vi "关键参数区.vi"(11 "数组":u16[](array[numeric]) format="%04xH") -> (3 "关键参数区":T1)   [LabVIEW 2016, in "斯坦道氨氮.lvlib"]
panel:
  # "共占用56 WORD"
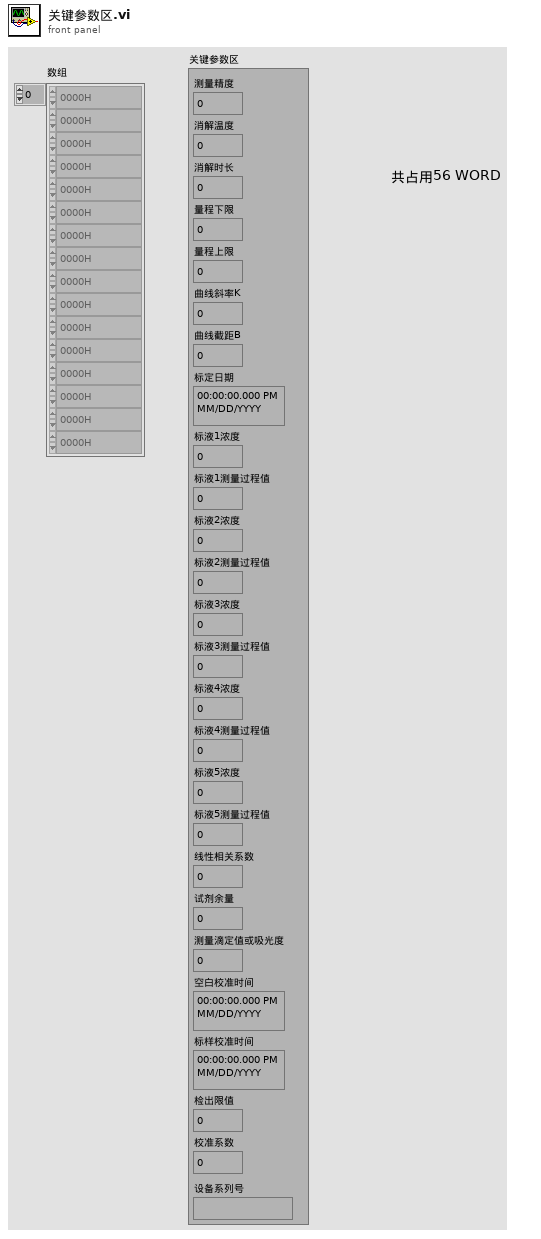
[diagram p1: front panel]
types:
  T1 = cluster{"测量精度":u16, "消解温度":u16, "消解时长":u16, "量程下限":sgl, "量程上限":sgl, "曲线斜率K":sgl, "曲线截距B":sgl, "标定日期":timestamp, "标液1浓度":sgl, "标液1测量过程值":sgl, "标液2浓度":sgl, "标液2测量过程值":sgl, "标液3浓度":sgl, "标液3测量过程值":sgl, "标液4浓度":sgl, "标液4测量过程值":sgl, "标液5浓度":sgl, "标液5测量过程值":sgl, "线性相关系数":sgl, "试剂余量":u32, "测量滴定值或吸光度":sgl, "空白校准时间":timestamp, "标样校准时间":timestamp, "检出限值":sgl, "校准系数":sgl, "设备系列号":string}
  T2 = cluster{"WORD":u16, "WORD":u16, "WORD":u16, "FLOAT":sgl, "FLOAT":sgl, "FLOAT":sgl, "FLOAT":sgl, "time stamp":timestamp, "FLOAT":sgl, "FLOAT":sgl, "FLOAT":sgl, "FLOAT":sgl, "FLOAT":sgl, "FLOAT":sgl, "FLOAT":sgl, "FLOAT":sgl, "FLOAT":sgl, "FLOAT":sgl, "FLOAT":sgl, "DWORD":i32, "FLOAT":sgl, "time stamp":timestamp, "time stamp":timestamp, "FLOAT":sgl, "FLOAT":sgl, "string":string}
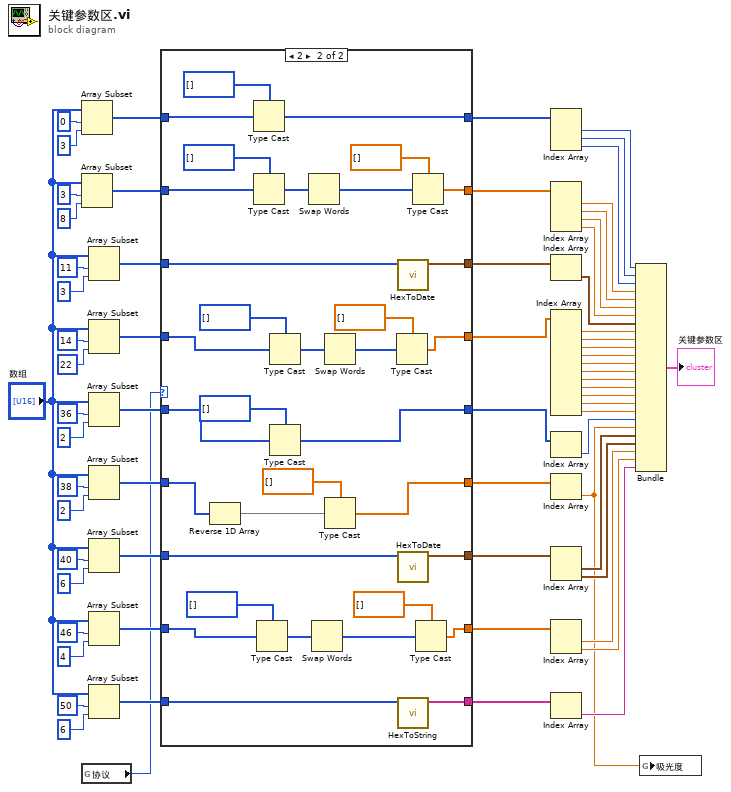
[diagram p0: block diagram]
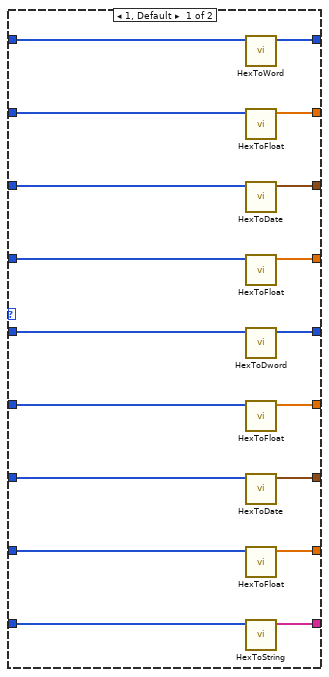
[diagram p2: hidden frame]
diagram:
  n1 = Array Subset(array="数组", index=0 ("索引"), length=3 ("长度")) -> (w60:u16[])
  n2 = Array Subset(array="数组", index=3 ("索引"), length=8 ("长度")) -> (w56:u16[])
  n3 = global read "总磷总氮断电保存全局变量.vi" "协议"() -> (w2:u16)
  n4 = Array Subset(array="数组", index=11 ("索引"), length=3 ("长度")) -> (w48:u16[])
  n5 = Array Subset(array="数组", index=14 ("索引"), length=22 ("长度")) -> (w43:u16[])
  n6 = Array Subset(array="数组", index=36 ("索引"), length=2 ("长度")) -> (w18:u16[])
  n7 = Array Subset(array="数组", index=38 ("索引"), length=2 ("长度")) -> (w19:u16[])
  n8 = Array Subset(array="数组", index=40 ("索引"), length=6 ("长度")) -> (w31:u16[])
  n9 = Array Subset(array="数组", index=46 ("索引"), length=4 ("长度")) -> (w26:u16[])
  n10 = Array Subset(array="数组", index=50 ("索引"), length=6 ("长度")) -> (w20:u16[])
  n11 = case shown="2" w2 {
    tunnel: w60 -> [w83 w85]
    tunnel: [w82 w84] -> w59
    tunnel: w56 -> [w81 w86]
    tunnel: [w80 w87] -> w55
    tunnel: w48 -> [w79 w117]
    tunnel: [w78 w116] -> w47
    tunnel: w43 -> [w77 w96]
    tunnel: [w76 w95] -> w42
    tunnel: [w75 w94] -> w37
    tunnel: w31 -> [w74 w115]
    tunnel: [w73 w114] -> w30
    tunnel: w26 -> [w72 w107]
    tunnel: [w71 w106] -> w24
    tunnel: w20 -> [w70 w113]
    tunnel: w19 -> [w69 w98]
    tunnel: w18 -> [w68 w97]
    tunnel: [w67 w93] -> w14
    tunnel: [w66 w112] -> w4
    frame 1, Default {
      n12 = call "HexToWord.vi"("数组"=w83) -> ("WORD"=w82:u16[])  [unwired: 10 in]
      n13 = call "HexToFloat.vi"("数组"=w81) -> ("FLOAT"=w80:sgl[])  [unwired: 10 in]
      n14 = call "HexToDate.vi"("数组"=w79) -> ("DATE"=w78:timestamp[])  [unwired: 10 in]
      n15 = call "HexToFloat.vi"("数组"=w77) -> ("FLOAT"=w76:sgl[])  [unwired: 10 in]
      n16 = call "HexToDword.vi"("数组"=w68) -> ("DWORD"=w75:i32[])  [unwired: 10 in]
      n17 = call "HexToFloat.vi"("数组"=w69) -> ("FLOAT"=w67:sgl[])  [unwired: 10 in]
      n18 = call "HexToDate.vi"("数组"=w74) -> ("DATE"=w73:timestamp[])  [unwired: 10 in]
      n19 = call "HexToFloat.vi"("数组"=w72) -> ("FLOAT"=w71:sgl[])  [unwired: 10 in]
      n20 = call "HexToString.vi"("数组"=w70) -> ("STRING"=w66:string[])  [unwired: 10 in]
    }
    frame 2 {
      n21 = Reverse 1D Array(array=w98) -> (reversed array=w100:u16[])
      n22 = Type Cast(type=u16[] [], x=w85) -> (*(type *) &x=w84:u16[])
      n23 = Type Cast(type=i32[] [], x=w86) -> (*(type *) &x=w90:i32[])
      n24 = Type Cast(type=i32[] [], x=w107) -> (*(type *) &x=w109:i32[])
      n25 = Type Cast(type=i32[] [], x=w96) -> (*(type *) &x=w104:i32[])
      n26 = Type Cast(type=u16[] [], x=w97) -> (*(type *) &x=w94:u16[])
      n27 = Swap Words(1:w90) -> (0:w88:i32[])
      n28 = Swap Words(1:w109) -> (0:w111:i32[])
      n29 = Swap Words(1:w104) -> (0:w102:i32[])
      n30 = Type Cast(type=sgl[] [], x=w100) -> (*(type *) &x=w93:sgl[])
      n31 = Type Cast(type=sgl[] [], x=w102) -> (*(type *) &x=w95:sgl[])
      n32 = call "HexToDate.vi"("数组"=w117) -> ("DATE"=w116:timestamp[])  [unwired: 10 in]
      n33 = call "HexToDate.vi"("数组"=w115) -> ("DATE"=w114:timestamp[])  [unwired: 10 in]
      n34 = call "HexToString.vi"("数组"=w113) -> ("STRING"=w112:string[])  [unwired: 10 in]
      n35 = Type Cast(type=sgl[] [], x=w88) -> (*(type *) &x=w87:sgl[])
      n36 = Type Cast(type=sgl[] [], x=w111) -> (*(type *) &x=w106:sgl[])
    }
  }
  n37 = Index Array(array=w59) -> (element #1=w63:u16, element #2=w62:u16, element #3=w61:u16)  [unwired: 3 in]
  n38 = Index Array(array=w55) -> (element #1=w54:sgl, element #2=w53:sgl, element #3=w52:sgl, element #4=w51:sgl)  [unwired: 4 in]
  n39 = Index Array(array=w47) -> (element=w46:timestamp)  [unwired: 1 in]
  n40 = Index Array(array=w42) -> (element #1=w41:sgl, element #2=w40:sgl, element #3=w39:sgl, element #4=w38:sgl, element #5=w12:sgl, element #6=w11:sgl, element #7=w10:sgl, element #8=w9:sgl, element #9=w8:sgl, element #10=w7:sgl, element #11=w6:sgl)  [unwired: 11 in]
  n41 = Index Array(array=w37) -> (element=w34:i32)  [unwired: 1 in]
  n42 = Index Array(array=w14) -> (element=w1:sgl)  [unwired: 1 in]
  n43 = Index Array(array=w30) -> (element #1=w29:timestamp, element #2=w28:timestamp)  [unwired: 2 in]
  n44 = Index Array(array=w24) -> (element #1=w23:sgl, element #2=w13:sgl)  [unwired: 2 in]
  n45 = Index Array(array=w4) -> (element=w3:string)  [unwired: 1 in]
  n46 = Bundle("WORD"=w63, "WORD"=w62, "WORD"=w61, "FLOAT"=w54, "FLOAT"=w53, "FLOAT"=w52, "FLOAT"=w51, "time stamp"=w46, "FLOAT"=w41, "FLOAT"=w40, "FLOAT"=w39, "FLOAT"=w38, "FLOAT"=w12, "FLOAT"=w11, "FLOAT"=w10, "FLOAT"=w9, "FLOAT"=w8, "FLOAT"=w7, "FLOAT"=w6, "DWORD"=w34, "FLOAT"=w1, "time stamp"=w29, "time stamp"=w28, "FLOAT"=w23, "FLOAT"=w13, "string"=w3) -> (→"关键参数区":T2)  [unwired: 1 in]
  n47 = global write "总磷总氮断电保存全局变量.vi" "吸光度"(w1) -> ()
